vi "Stop loop.vi"(5 "Loop iteration (ms)":u32=3000) -> (2 "Stop":bool)   [LabVIEW 2013]
uses:
  Global Variables/General Globals.vi
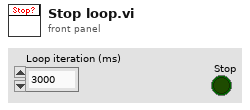
[diagram p1: front panel]
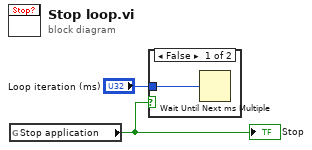
[diagram p0: block diagram]
diagram:
  n1 = global read "General Globals.vi" "Stop application"() -> (w2:bool)
  "Stop" <- w2
  n2 = case shown="False" w2 {
    tunnel: "Loop iteration (ms)" -> [w3 _]
    frame False {
      n3 = Wait Until Next ms Multiple(millisecond multiple=w3) -> ()  [unwired: 1 out]
    }
    frame True {
    }
  }
